vi "Read Config Data.vi"(8 "Error In":errorcluster, 11 "configuration file in":path) -> (0 "Error Out":errorcluster, 2 "Hardware Settings":T1={"AI Voltage Channel"="PCI-6221/ai0", "Sample Rate (Hz)"=1000.0, "Samples per channel"=1000, "AO Voltage Channel"="PCI-6221/ao1"}, 3 "configuration file out":path)   [LabVIEW 2020]
uses:
  Hardware Settings.ctl
  <vilib>/Utility/config.llb/Read Key (String).vi
  <vilib>/Utility/config.llb/Read Key (Double).vi
  <vilib>/Utility/config.llb/Read Key (I32).vi
  <vilib>/Utility/config.llb/NI_LVConfig.lvlib
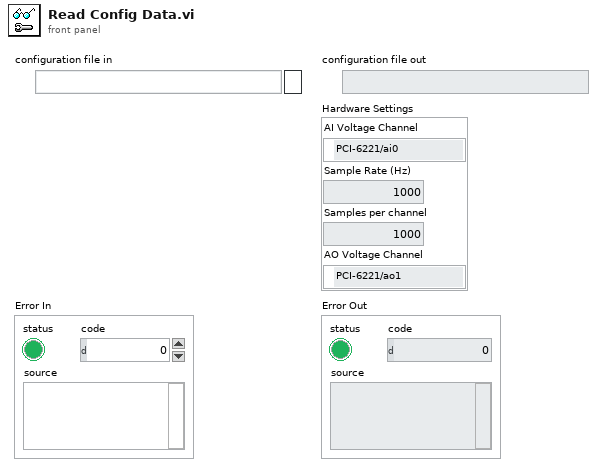
[diagram p1: front panel]
types:
  T1 = typedef "Hardware Settings.ctl" = cluster{"AI Voltage Channel":tag, "Sample Rate (Hz)":dbl, "Samples per channel":i32, "AO Voltage Channel":tag}
  T2 = typedef "NI_LVConfig.lvlib/Config Data RefNum.ctl" = refnum<k1>
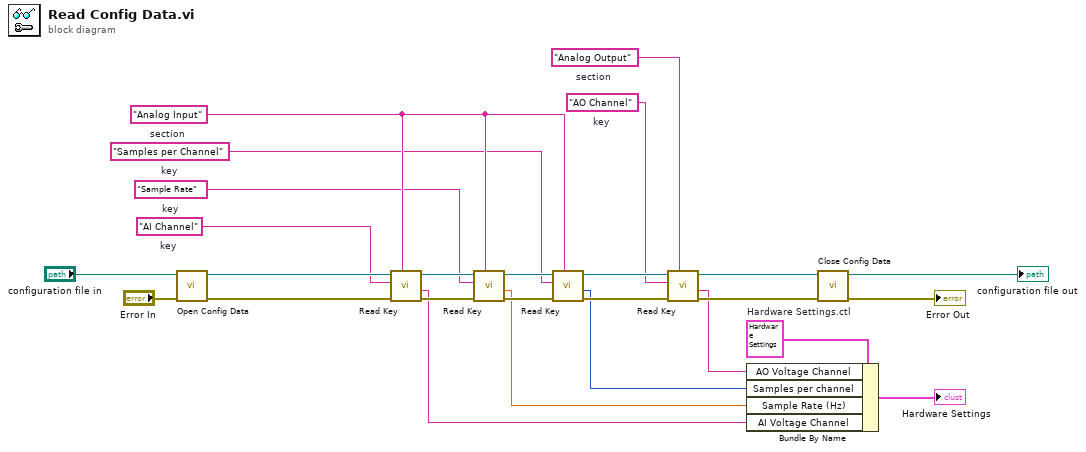
[diagram p0: block diagram]
diagram:
  w6 = T1 {"AI Voltage Channel"="PCI-6221/ai0", "Sample Rate (Hz)"=1000.0, "Samples per channel"=1000, "AO Voltage Channel"="PCI-6221/ao1"}  # Hardware Settings.ctl
  w7 = "Analog Output"  # section
  w21 = "Analog Input"  # section
  w8 = "AO Channel"  # key
  w9 = "Samples per Channel"  # key
  w10 = "Sample Rate"  # key
  w22 = "AI Channel"  # key
  n1 = call <vilib>:"Open Config Data.vi"("error in (no error)"="Error In", "configuration file path"="configuration file in") -> ("error out"=w23:errorcluster, "refnum"=w24:T2)  [unwired: 7 in, 1 out]
  n2 = call-poly <vilib>:"Read Key.vi"("section"=w21, "error in (no error)"=w23, "key"=w22, "refnum"=w24) -> ("error out"=w17:errorcluster, "value"=w2:string, "refnum out"=w20:T2)  [unwired: 4 in, 1 out]
  n3 = call-poly <vilib>:"Read Key.vi"("section"=w21, "error in (no error)"=w17, "key"=w10, "refnum"=w20) -> ("error out"=w16:errorcluster, "value"=w3:dbl, "refnum out"=w19:T2)  [unwired: 4 in, 1 out]
  n4 = call-poly <vilib>:"Read Key.vi"("section"=w21, "error in (no error)"=w16, "key"=w9, "refnum"=w19) -> ("error out"=w15:errorcluster, "value"=w4:i32, "refnum out"=w18:T2)  [unwired: 4 in, 1 out]
  n5 = call-poly <vilib>:"Read Key.vi"("section"=w7, "error in (no error)"=w15, "key"=w8, "refnum"=w18) -> ("error out"=w14:errorcluster, "value"=w5:string, "refnum out"=w13:T2)  [unwired: 4 in, 1 out]
  n6 = Bundle By Name(cluster=w6, "AO Voltage Channel"=w5, "Samples per channel"=w4, "Sample Rate (Hz)"=w3, "AI Voltage Channel"=w2) -> (→"Hardware Settings":T1)
  n7 = call <vilib>:"Close Config Data.vi"("error in (no error)"=w14, "refnum"=w13) -> ("error out"=→"Error Out":errorcluster, "file path"=→"configuration file out":path)  [unwired: 8 in]
